vi "AI data read.vi"(8 "error in":errorcluster, 11 "Message Queues in":T3) -> (0 "error out":errorcluster, 3 "NI Analog Input":T1 {"Analog Result"."Számolt NTC hõmérséklet" format="%.3g"; "Analog Result"."15V" format="%.3g"; "Analog Result"."Elvárt NTC ellenállás" format="%.3g"; "Analog Result"."48V" format="%.3g"; "Analog Result"."Hõmérséklet" format="%.3g"; "Analog Result"."Szigetelési ellenállás" format="%.3g"; "Analog Result"."NTC ellenállás" format="%.3g"; "Analog Result"."Szenzor ellenállás" format="%.3g"})   [LabVIEW 2014]
uses:
  support/Message Queue/All Message Queues.ctl
  support/Message Queue/Message Cluster.ctl
  Analog Input Cluster.ctl
  Analog Result Cluster.ctl
  support/Message Queue/Message Queue.lvlib
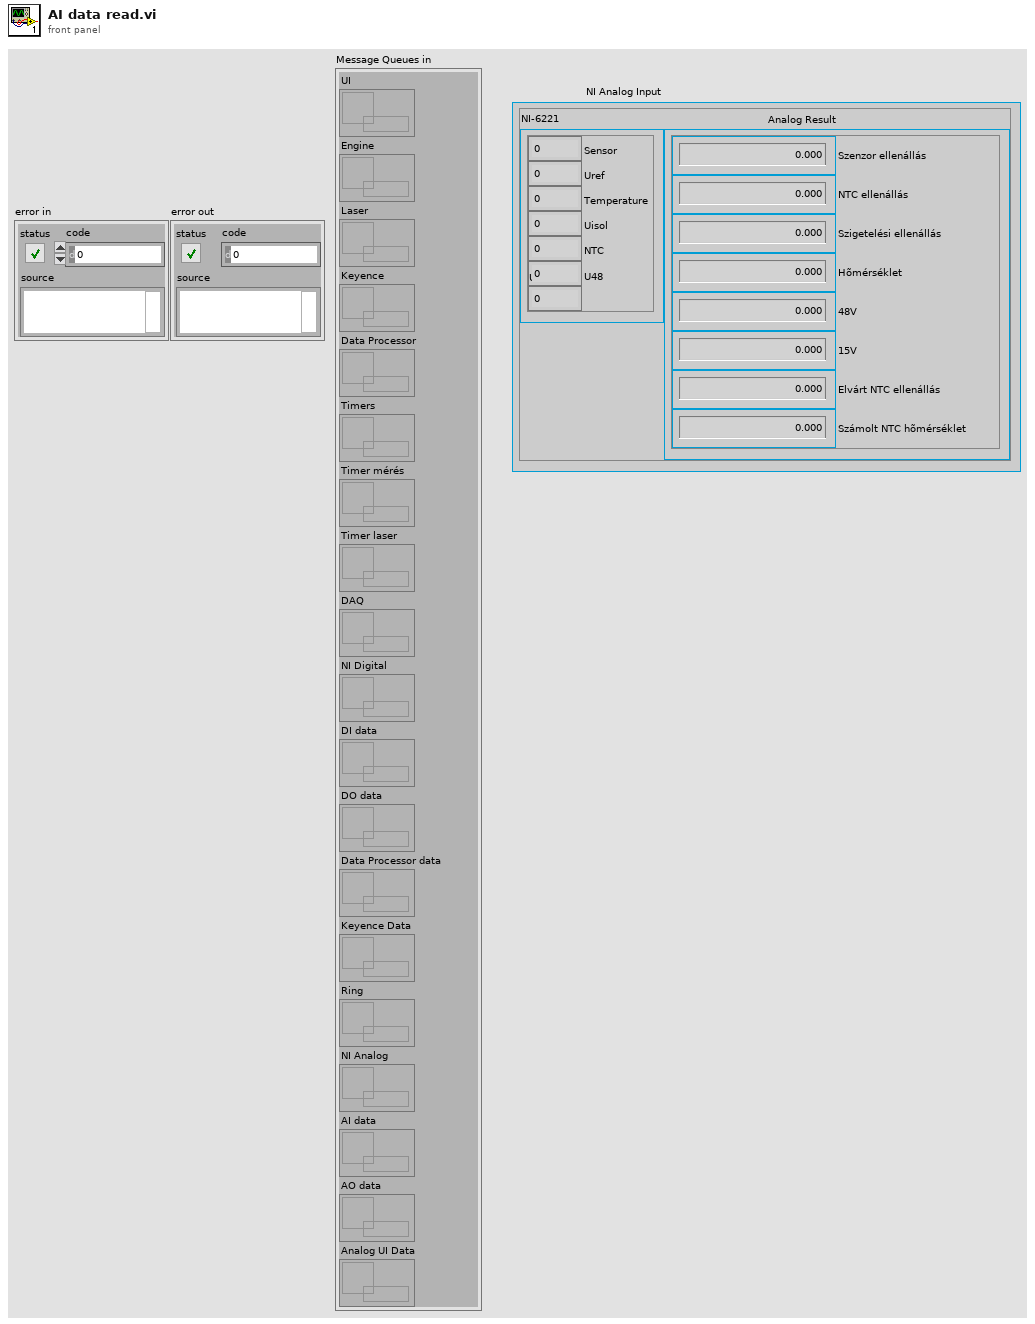
[diagram p1: front panel]
types:
  T1 = typedef "Analog Input Cluster.ctl" = cluster{"NI-6221":cluster{"Sensor":dbl, "Uref":dbl, "Temperature":dbl, "Uisol":dbl, "NTC":dbl, "U48":dbl, "U15":dbl}, "Analog Result":T2}
  T2 = typedef "Analog Result Cluster.ctl" = cluster{"Szenzor ellenállás":dbl, "NTC ellenállás":dbl, "Szigetelési ellenállás":dbl, "Hõmérséklet":dbl, "48V":dbl, "15V":dbl, "Elvárt NTC ellenállás":dbl, "Számolt NTC hõmérséklet":dbl}
  T3 = typedef "Message Queue.lvlib/All Message Queues.ctl" = cluster{"UI":refnum<queue>, "Engine":refnum<queue>, "Laser":refnum<queue>, "Keyence":refnum<queue>, "Data Processor":refnum<queue>, "Timers":refnum<queue>, "Timer mérés":refnum<queue>, "Timer laser":refnum<queue>, "DAQ":refnum<queue>, "NI Digital":refnum<queue>, "DI data":refnum<queue>, "DO data":refnum<queue>, "Data Processor data":refnum<queue>, "Keyence Data":refnum<queue>, "Ring":refnum<queue>, "NI Analog":refnum<queue>, "AI data":refnum<queue>, "AO data":refnum<queue>, "Analog UI Data":refnum<queue>}
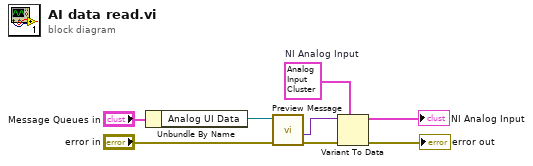
[diagram p0: block diagram]
diagram:
  w3 = T1 {"NI-6221"={"Sensor"=0.0, "Uref"=0.0, "Temperature"=0.0, "Uisol"=0.0, "NTC"=0.0, "U48"=0.0, "U15"=0.0}, "Analog Result"={"Szenzor ellenállás"=0.0, "NTC ellenállás"=0.0, "Szigetelési ellenállás"=0.0, "Hõmérséklet"=0.0, "48V"=0.0, "15V"=0.0, "Elvárt NTC ellenállás"=0.0, "Számolt NTC hõmérséklet"=0.0}}  # NI Analog Input
  n1 = Unbundle By Name("Message Queues in") -> ("Analog UI Data"=w7:refnum<queue>)
  n2 = call "Preview Message.vi"("error in (no error)"="error in", "Message Queue"=w7) -> ("error out"=w6:errorcluster, "Message Data"=w5:variant)  [unwired: 5 in, 3 out]
  n3 = Variant To Data(error in=w6, type=w3, Variant=w5) -> (data=→"NI Analog Input":T1, error out=→"error out":errorcluster)
